vi "Save Report to Database.vi"(0 "barcode":string, 1 "Input":string[](array[string]), 2 "Option":enum16{"Write", "Log", "Log Barcode"}(ring), 5 "modelid":string, 7 "varintid":string, 9 "stationid":string, 11 "error in (no error)":errorcluster) -> (15 "error out":errorcluster)   [LabVIEW 2020]
uses:
  Database/Controls/DB Options.ctl
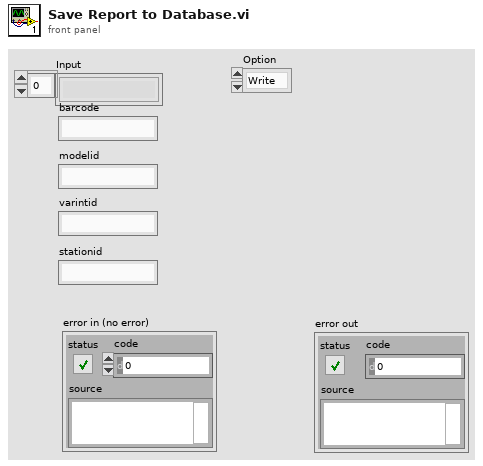
[diagram p1: front panel]
types:
  T1 = cluster{"modelid":string, "varintid":string, "stationid":string, "barcode":string}
  T2 = typedef "DB Options.ctl" = enum16{"Select", "Execute", "Special Q", "Insert", "Update", "Delete", "Open", "Close"}
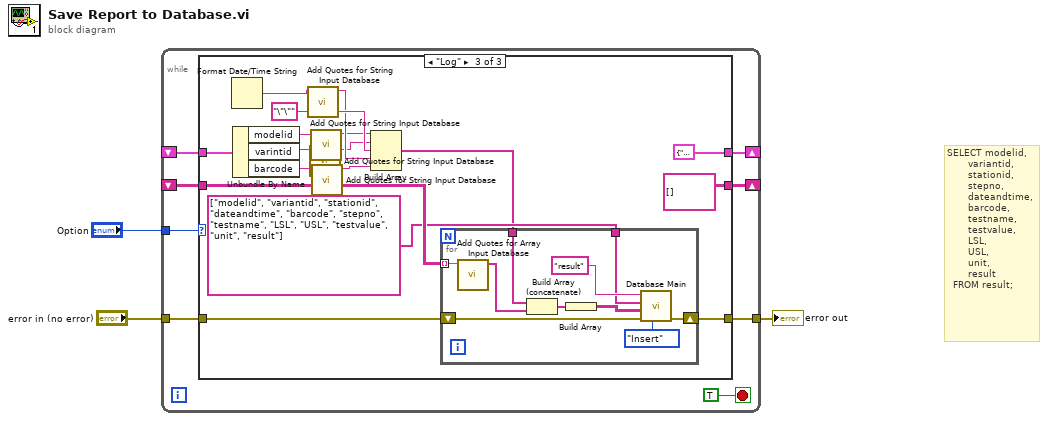
[diagram p0: block diagram]
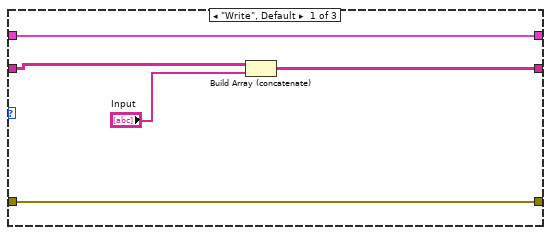
[diagram p2: hidden frame]
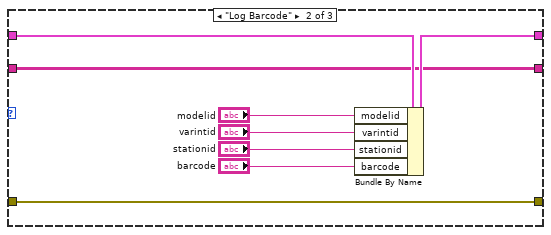
[diagram p3: hidden frame]
diagram:
  # "SELECT modelid,\n       variantid,\n       stationid,\n       stepno,\n       dateandtime,\n       barcode,\n       testname,\n       testvalue,\n       LSL,\n       USL,\n       unit,\n       result\n  FROM result;"
  n1 = while {
    tunnel: "Option" -> [w11]
    shift-right: [w10] -> _
    shift-left: _ -> [w9]
    tunnel: "error in (no error)" -> [w7]
    tunnel: [w6] -> w1
    shift-right: [w5] -> _
    shift-left: _ -> [w4]
    stop <- TRUE stop-if-true
    n2 = case shown="\"Log\"" w11 {
      tunnel: [w15 w17 string[][] []] -> w10
      tunnel: w9 -> [w14 w17 w38]
      tunnel: w7 -> [w13 w24 w40]
      tunnel: [w13 w24 w39] -> w6
      tunnel: [w12 w22 T1 {"modelid"="", "varintid"="", "stationid"="", "barcode"=""}] -> w5
      tunnel: w4 -> [w12 w23 w35]
      frame "Write", Default {
        n3 = Build Array (concatenate)(w14, "Input") -> (w15:string[][])
      }
      frame "Log Barcode" {
        n4 = Bundle By Name(cluster=w23, "modelid"="modelid", "varintid"="varintid", "stationid"="stationid", "barcode"="barcode") -> (w22:T1)
      }
      frame "Log" {
        n5 = Format Date/Time String() -> (date/time string=w30:string)  [unwired: 3 in]
        n6 = Unbundle By Name(w35) -> ("modelid"=w27:string, "varintid"=w26:string, "barcode"=w34:string)
        n7 = call "Add Quotes for String Input Database.vi"("String in"=w30) -> ("String Out"=w29:string)  [unwired: 10 in]
        n8 = call "Add Quotes for String Input Database.vi"("String in"=w26) -> ("String Out"=w25:string)  [unwired: 10 in]
        n9 = call "Add Quotes for String Input Database.vi"("String in"=w27) -> ("String Out"=w28:string)  [unwired: 10 in]
        n10 = call "Add Quotes for String Input Database.vi"("String in"=w34) -> ("String Out"=w33:string)  [unwired: 10 in]
        n11 = Build Array(w28, w25, "\"\"" ("element"), w29, w33) -> (w32:string[])
        n12 = for {
          shift-right: [w49] -> w39
          shift-left: w40 -> [w50]
          tunnel: w38 -> [w48] mode=indexing
          tunnel: string[] ["modelid", "variantid", "stationid", "dateandtime", "barcode", "stepno", "testname", "LSL", "USL", "testvalue", "unit", "result"] ("Column Name") -> [w45]
          tunnel: w32 -> [w44]
          n13 = call "Add Quotes for Array Input Database.vi"("Array Input"=w48) -> ("Array Out"=w43:string[])  [unwired: 10 in]
          n14 = Build Array (concatenate)(w44, w43) -> (w47:string[])
          n15 = Build Array(w47) -> (w42:string[][])
          n16 = call "Database Main.vi"("Option"=DB_Options."Insert", "error in (no error)"=w50, "Column Values"=w42, "Column Name"=w45, "table Name/Query"="result") -> ("error out"=w49:errorcluster)  [unwired: 4 in, 2 out]
        }
      }
    }
  }
  "error out" <- w1
